vi "Logger Close Queuey.vi"(11 "error in (no error)":errorcluster) -> (15 "error out":errorcluster)   [LabVIEW 2018]
uses:
  Logger Global.vi
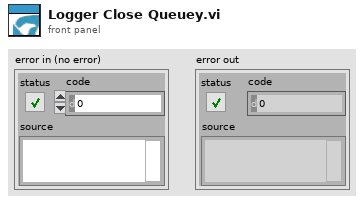
[diagram p1: front panel]
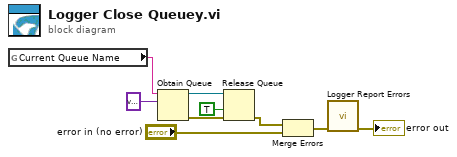
[diagram p0: block diagram]
diagram:
  n1 = global read "Logger Global.vi" "Current Queue Name"() -> (w4:string)
  n2 = Obtain Queue(name (unnamed)=w4, element data type=variant) -> (queue out=w5:refnum<queue>, error out=w6:errorcluster)  [unwired: 3 in, 1 out]
  n3 = Release Queue(queue=w5, force destroy? (F)=TRUE, error in (no error)=w6) -> (error out=w8:errorcluster)  [unwired: 2 out]
  n4 = Merge Errors(w8, "error in (no error)") -> (w1:errorcluster)
  n5 = call "Logger Report Errors.vi"("error in (no error)"=w1) -> ("error out"=→"error out":errorcluster)  [unwired: 14 in]
